vi "create.vi"(10 "prefixTreeDelimiter":string) -> (3 "channelConfig":refnum<class "channelConfig.lvclass">)   [LabVIEW 2020, in "nominal types.lvlib" / "channelConfig.lvclass"]
uses:
  channelConfig.lvclass
  channelConfig.lvclass/channelConfig.ctl
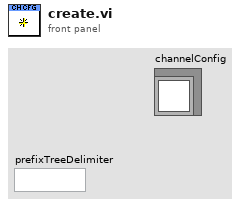
[diagram p1: front panel]
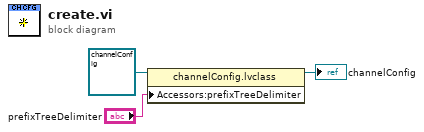
[diagram p0: block diagram]
diagram:
  n1 = property class="channelConfig.lvclass"(reference=refnum<class "channelConfig.lvclass"> refnum ("channelConfig in"), "Accessors:prefixTreeDelimiter"="prefixTreeDelimiter") -> (reference out=→"channelConfig":refnum<class "channelConfig.lvclass">)  [unwired: 1 in, 1 out]
